vi "wait on errorwire.vi"(4 "clear error?":bool, 6 "Delay Time (s)":dbl=1.0, 8 "error in (no error)":errorcluster) -> (0 "error out":errorcluster)   [LabVIEW 2012]
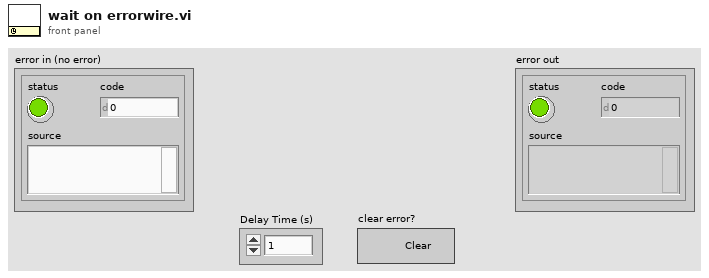
[diagram p1: front panel]
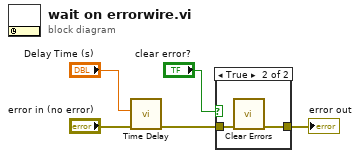
[diagram p0: block diagram]
diagram:
  n1 = call "Time Delay"("error in (no error)"="error in (no error)", "Delay Time (s)"="Delay Time (s)") -> ("error out"=w2:errorcluster)  [unwired: 9 in]
  n2 = case shown="True" "clear error?" {
    tunnel: w2 -> [w6 w8]
    tunnel: [w6 w7] -> w1
    frame False {
    }
    frame True {
      n3 = call <vilib>:"Clear Errors.vi"("error in (no error)"=w8) -> ("error out"=w7:errorcluster)  [unwired: 6 in]
    }
  }
  "error out" <- w1
